vi "VirtualPowerPlantWithModelBasedFaultDetection(Giulio_v1).vi"() -> ()   [LabVIEW 2017]
uses:
  <vilib>/Platform/TimedLoop/XDataNode/timing_clust.ctl
  <vilib>/Platform/TimedLoop/XDataNode/nitl_modes.ctl
  <vilib>/Platform/TimedLoop/XDataNode/wakeup.ctl
  <vilib>/Utility/file.llb/Write Delimited Spreadsheet (string).vi
  <vilib>/Utility/file.llb/Write Delimited Spreadsheet (DBL).vi
  <vilib>/platform/TimedLoop/XDataNode/XDataNode.xnode
  <vilib>/express/express arith-compare/Formula/XNode/ExpressFormulaBlockNode.xnode
  <vilib>/Platform/TimedLoop/XDataNode/XDNodeRunTimeDep.lvlib
panel:
  out "Sensor 4":cluster{"placeholder1":dbl, dbl}(graph)
  out "Sensor 3":cluster{"placeholder1":dbl, dbl}(graph)
  out "Sensor 2":cluster{"placeholder1":dbl, dbl}(graph)
  out "Sensor 1":cluster{"placeholder1":dbl, dbl}(graph)
  in  "dTsamplethreshold":dbl=10.0
  in  "Tsamplethreshold":dbl=3.0
  in  "dTthreshold4":dbl=2.1702
  in  "dTthreshold3":dbl=2.8362
  in  "dTthreshold2":dbl=2.6736
  in  "dTthreshold1":dbl=2.361
  in  "Tthreshold4":dbl=0.4812
  in  "Tthreshold3":dbl
  in  "Tthreshold2":dbl=0.5934
  in  "Tthreshold1":dbl=0.588
  in  "Weight of measured values in filter":dbl=0.01
  in  "CTAH_control_on":dbl
  in  "CTAH_setpoint":dbl
  in  "CTAH_freq":dbl
  in  "P_in":dbl
  in  "T_wall placeholder":dbl
  in  "mdot":dbl
  out "Warnings":string
  in  "stop":bool
  in  "Measured Values":dbl
  out "Cold Leg Temp":dbl
  out "Primary HX Outlet Temp":dbl
  out "Hot Leg Temp":dbl
  out "color3":u32(colorbox)
  out "Heater Outlet Temp":dbl caption="C"
  out "color4":u32(colorbox)
  out "color2":u32(colorbox)
  in  "Upper Operating Pressure":dbl=6154480.5
  in  "Pump Efficiency":dbl=0.95
  in  "Turbine Efficiency":dbl=0.95
  in  "Pinch Point Temp Difference":dbl=15.0
  in  "Lower Operating Pressure":dbl=7093.0
  in  "Mass Flowrate":dbl=418.0
  in  "Pressure Drop in HX 2nd pass":dbl
  in  "Pressure Drop in HX 1st pass":dbl
  in  "LPT Work Output":dbl=137940000.0
  in  "HPT Work Output":dbl=1000000.0
  in  "LPT Efficiency":dbl=0.8
  in  "HPT Efficiency":dbl=0.8
  in  "Compressor Efficiency":dbl=0.7
  in  "LPT Expansion Ratio":dbl=5.13
  in  "Incoming Air Pressure":dbl=101325.0
  in  "HPT Expansion Ratio":dbl=3.77
  in  "Incoming Air Temp":dbl=298.0
  in  "Compression Ratio":dbl=19.6
  out "h_1":dbl
  out "R_T_1":dbl
  out "R_P_1":dbl
  out "h_6":dbl
  out "R_T_6":dbl
  out "R_P_6":dbl
  out "h_5":dbl
  out "R_T_5":dbl
  out "R_P_5":dbl
  out "h_4":dbl
  out "R_T_4":dbl
  out "R_P_4":dbl
  out "T_6":dbl
  out "P_6":dbl
  out "T_5":dbl
  out "P_5":dbl
  out "T_4":dbl
  out "P_4":dbl
  out "T_3":dbl
  out "P_3":dbl
  out "T_2":dbl
  out "P_2":dbl
  out "T_1":dbl
  out "P_1":dbl
  out "color1":u32(colorbox)
  # "Reactor Loop"
  # "Brayton Cycle"
  # "Rankine Cycle"
  # "ST"
  # "Compressor"
  # "HPT"
  # "LPT"
  # "Reactor"
  # "HRSG"
  # "Primary Heat\nExchanger"
  # "Condenser"
  # "Pump"
  # "Pump"
  # "Developer's Tools"
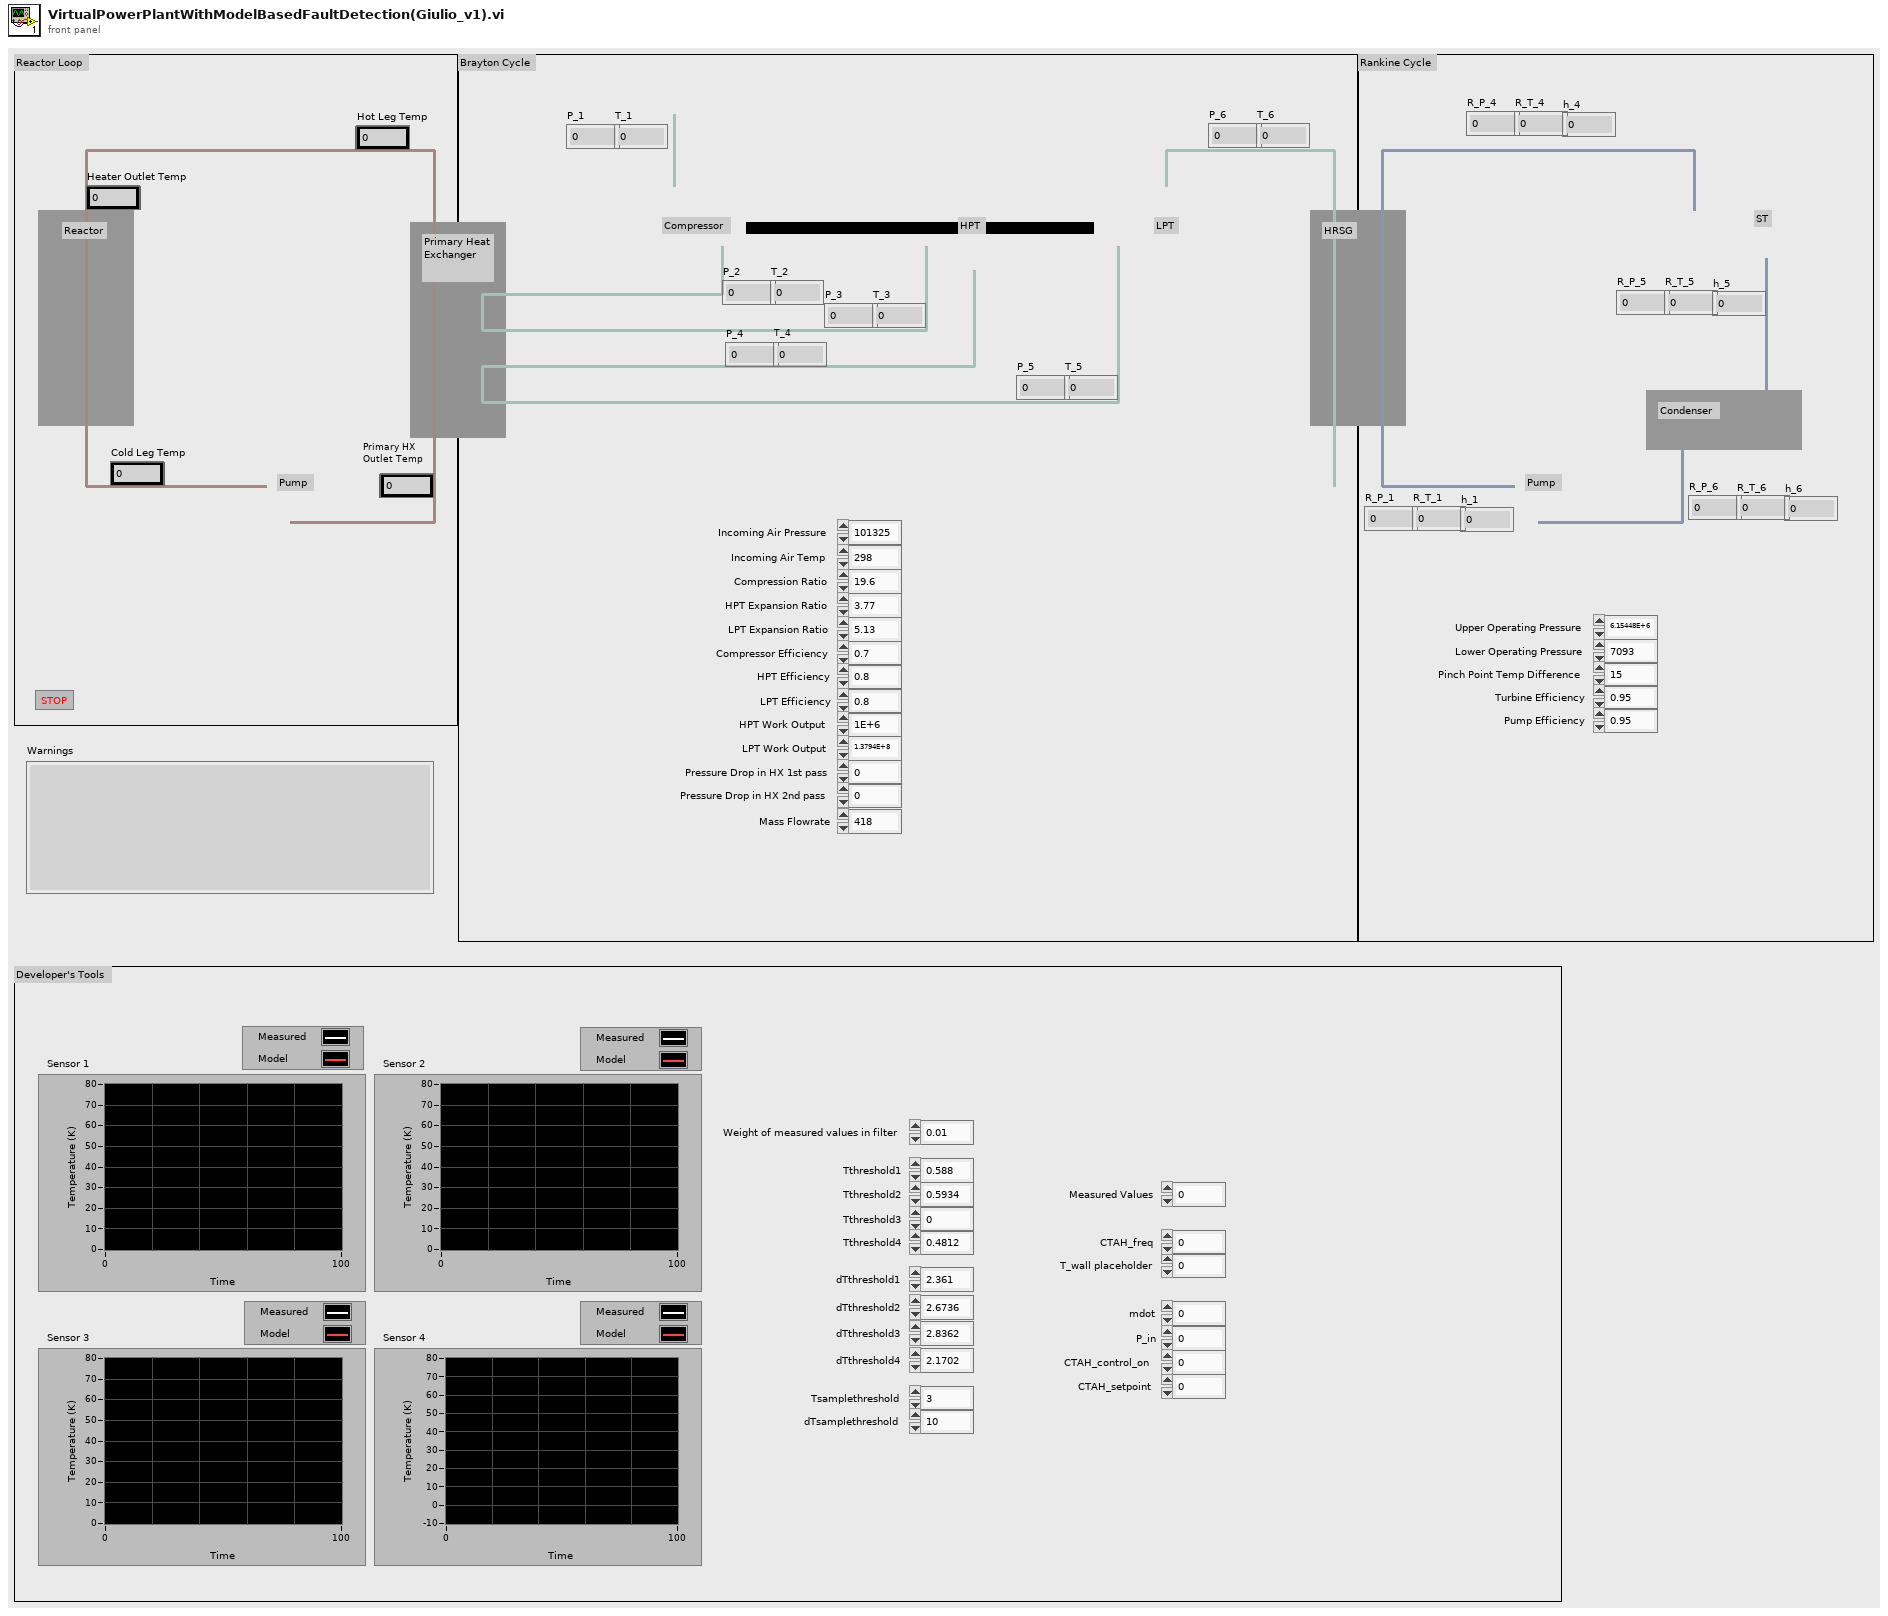
[diagram p1: front panel]
types:
  T1 = typedef "XDNodeRunTimeDep.lvlib/timing_clust.ctl" = cluster{"Expected End [f-1]":u64, "Actual End [f-1]":u64, "Finished Late? [f-1]":bool, "Expected End [i-1]":u64, "Actual End [i-1]":u64, "Finished Late? [i-1]":bool, "Expected Start [i]":u64, "Actual Start [i]":u64, "Expected Start [f]":u64, "Actual Start [f]":u64, "Source Name":string, "Structure Name":string, "Period":i64, "Deadline":i64, "Offset":i64, "Start":i64, "Priority":i32, "Timeout":i32, "Mode":T2, "Wakeup Reason":T3, "Error":errorcluster, "Source Type":string, "Secondary Source Type":string, "Global End Time":u64, "Global Start Time":u64, "Frame Duration":u64, "Iteration Duration":u64, "Assigned CPU":i32, "I/O Scan Engine Mode":u32}
  T2 = typedef "XDNodeRunTimeDep.lvlib/nitl_modes.ctl" = enum32{"No Change", "Process missed periods, maintain original phase", "Discard missed periods, maintain original phase", "Process missed periods, ignore original phase", "Discard missed periods, ignore original phase"}
  T3 = typedef "XDNodeRunTimeDep.lvlib/wakeup.ctl" = enum32{"Normal", "Aborted", "Asynchronous wakeup", "Timing source error", "Timed loop error", "Timeout"}
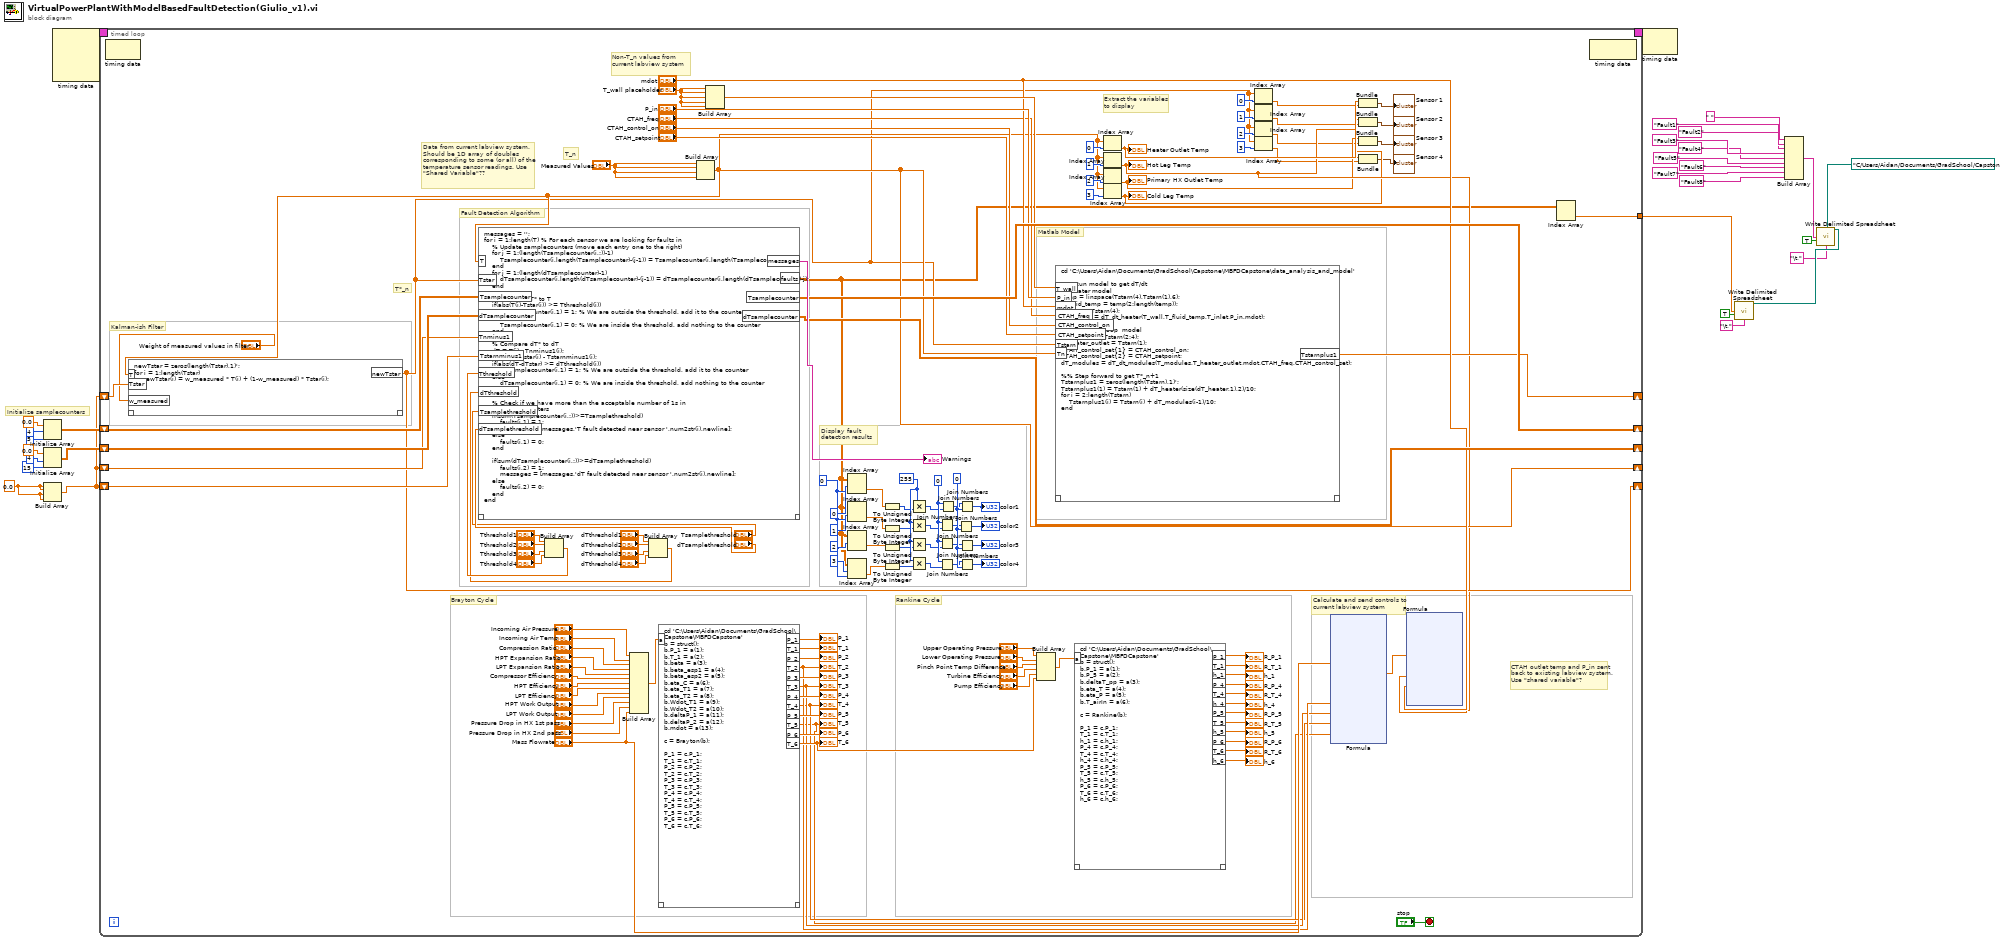
[diagram p0: block diagram]
diagram:
  w19 = 0.0
  # "Initialize samplecounters"
  n1 = Initialize Array(0.0, 4, 5) -> (w25:dbl[][])
  n2 = Initialize Array(0.0, 4, 15) -> (w24:dbl[][])
  n3 = Build Array(w19, w19, w19, w19) -> (w18:dbl[])
  n4 = node-c288() -> (w29:T1)  [unwired: 4 in]
  n5 = timed-loop {
    shift-right: [w93] -> _
    shift-left: w18 -> [w92]
    shift-right: [w105] -> _
    shift-left: w25 -> [w103]
    shift-right: [w104] -> _
    shift-left: w24 -> [w102]
    shift-right: [w91] -> _
    shift-left: w18 -> [w101]
    shift-right: [w44] -> _
    shift-left: w18 -> [w100]
    timing: w29 -> [_]
    timing-out: [_] -> w28
    tunnel: [w30] -> w17
    stop <- "stop" stop-if-true
    w61 = u8 255
    w62 = u8 0
    w63 = u8 0
    w68 = 0
    # "Kalman-ish Filter"
    # "Non-T_n values from current labview system"
    # "Extract the variables to display"
    # "T_n"
    # "Data from current labview system. Should be 1D array of doubles corresponding to some (or all) of the temperature sensor readings. Use \"Shared Variable\"??"
    # "CTAH outlet temp and P_in sent back to existing labview system. Use \"shared variable\"?"
    # "Calculate and send controls to current labview system"
    # "Display fault detection results"
    # "Fault Detection Algorithm"
    # "T*_n"
    # "Matlab Model"
    # "Rankine Cycle"
    # "Brayton Cycle"
    n6 = node-c288() -> ()  [unwired: 1 in, 1 out]
    n7 = Build Array("Tthreshold1", "Tthreshold2", "Tthreshold3", "Tthreshold4") -> (w85:dbl[])
    n8 = Build Array("Incoming Air Pressure", "Incoming Air Temp", "Compression Ratio", "HPT Expansion Ratio", "LPT Expansion Ratio", "Compressor Efficiency", "HPT Efficiency", "LPT Efficiency", "HPT Work Output", "LPT Work Output", "Pressure Drop in HX 1st pass", "Pressure Drop in HX 2nd pass", "Mass Flowrate") -> (w145:dbl[])
    n9 = Build Array("dTthreshold1", "dTthreshold2", "dTthreshold3", "dTthreshold4") -> (w80:dbl[])
    n10 = script code="cd 'C:\\Users\\Aidan\\Documents\\GradSchool\\Capstone\\MBFDCapstone'\nb = struct();\nb.P_1 = a(1);\nb.T_1 = a(2);\nb.beta = a(3);\nb.beta_esp1 = a(4);\nb.beta_esp2 = a(5);\nb.eta_C = a(6);\nb.eta_T1 = a(7);\nb.eta_T2 = a(8);\nb.Wdot_T1 = a(9);\nb.Wdot_T2 = a(10);\nb.deltaP_1 = a(11);\nb.deltaP_2 = a(12);\nb.mdot = a(13);\n\nc = Brayton(b);\n\nP_1 = c.P_1;\nT_1 = c.T_1;\nP_2 = c.P_2;\nT_2 = c.T_2;\nP_3 = c.P_3;\nT_3 = c.T_3;\nP_4 = c.P_4;\nT_4 = c.T_4;\nP_5 = c.P_5;\nT_5 = c.T_5;\nP_6 = c.P_6;\nT_6 = c.T_6;"("a"=w145) -> ("P_1"=→"P_1":dbl, "T_1"=→"T_1":dbl, "P_2"=→"P_2":dbl, "T_2"=w110:dbl, "P_3"=→"P_3":dbl, "T_3"=w109:dbl, "P_4"=→"P_4":dbl, "T_4"=w108:dbl, "P_5"=→"P_5":dbl, "T_5"=w107:dbl, "P_6"=→"P_6":dbl, "T_6"=w131:dbl)  [unwired: 1 in, 1 out]
    "T_2" <- w110
    "T_3" <- w109
    "T_4" <- w108
    "T_5" <- w107
    "T_6" <- w131
    n11 = Build Array("Measured Values", "Measured Values", "Measured Values", "Measured Values") -> (w91:dbl[])
    n12 = script code="newTstar = zeros(length(Tstar),1)';\nfor i = 1:length(Tstar)\n    newTstar(i) = w_measured * T(i) + (1-w_measured) * Tstar(i);\nend"("T"=w91, "Tstar"=w92, "w_measured"="Weight of measured values in filter") -> ("newTstar"=w44:dbl[])  [unwired: 1 in, 1 out]
    n13 = script code="messages = '';\nfor i = 1:length(T) % For each sensor we are looking for faults in\n    % Update samplecounters (move each entry one to the right)\n    for j = 1:(length(Tsamplecounter(i,:))-1)\n        Tsamplecounter(i,length(Tsamplecounter)-(j-1)) = Tsamplecounter(i,length(Tsamplecounter)-j);\n    end\n    for j = 1:(length(dTsamplecounter)-1)\n        dTsamplecounter(i,length(dTsamplecounter)-(j-1)) = dTsamplecounter(i,length(dTsamplecounter)-j);\n    end\n\n    % Compare T* to T\n    if(abs(T(i)-Tstar(i)) >= Tthreshold(i))\n        Tsamplecounter(i,1) = 1; % We are outside the threshold, add it to the counter\n    else\n        Tsamplecounter(i,1) = 0; % We are inside the threshold, add nothing to the counter\n    end\n    \n    % Compare dT* to dT\n    dT = T(i) - Tnminus1(i);\n    dTstar = Tstar(i) - Tstarnminus1(i);\n    if(abs(dT-dTstar) >= dTthreshold(i))\n        dTsamplecounter(i,1) = 1; % We are outside the threshold, add it to the counter\n    else\n        dTsamplecounter(i,1) = 0; % We are inside the threshold, add nothing to the counter\n    end\n    \n    % Check if we have more than the acceptable number of 1s in\n    % samplecounters\n    if(sum(Tsamplecounter(i,:))>=Tsamplethreshold)\n        faults(i,1) = 1;\n        messages = [messages,'T fault detected near sensor ',num2str(i),newline];\n    else\n        faults(i,1) = 0;\n    end\n       \n    if(sum(dTsamplecounter(i,:))>=dTsamplethreshold)\n        faults(i,2) = 1;\n        messages = [messages,'dT fault detected near sensor ',num2str(i),newline];\n    else\n        faults(i,2) = 0;\n    end\nend"("T"=w91, "Tstar"=w44, "Tsamplecounter"=w103, "dTsamplecounter"=w102, "Tnminus1"=w101, "Tstarnminus1"=w100, "Tthreshold"=w85, "dTthreshold"=w80, "Tsamplethreshold"="Tsamplethreshold", "dTsamplethreshold"="dTsamplethreshold") -> ("faults"=w31:dbl[][], "messages"=→"Warnings":string, "Tsamplecounter"=w105:dbl[][], "dTsamplecounter"=w104:dbl[][])  [unwired: 1 in, 1 out]
    n14 = Build Array("T_wall placeholder", "T_wall placeholder", "T_wall placeholder", "T_wall placeholder", "T_wall placeholder") -> (w99:dbl[])
    n15 = Index Array(array=w31, index (row)=0, index (col)=w68) -> (element=w64:dbl)
    n16 = Index Array(array=w31, index (row)=1, index (col)=w68) -> (element=w65:dbl)
    n17 = Index Array(array=w31, index (row)=2, index (col)=w68) -> (element=w66:dbl)
    n18 = Index Array(array=w31, index (row)=3, index (col)=w68) -> (element=w67:dbl)
    n19 = To Unsigned Byte Integer(number=w64) -> (unsigned 8bit integer=w60:u8)
    n20 = To Unsigned Byte Integer(number=w65) -> (unsigned 8bit integer=w58:u8)
    n21 = To Unsigned Byte Integer(number=w66) -> (unsigned 8bit integer=w56:u8)
    n22 = To Unsigned Byte Integer(number=w67) -> (unsigned 8bit integer=w54:u8)
    n23 = Multiply(x=w61, y=w60) -> (x*y=w59:u8)
    n24 = Multiply(x=w61, y=w58) -> (x*y=w57:u8)
    n25 = Multiply(x=w61, y=w56) -> (x*y=w55:u8)
    n26 = Multiply(x=w61, y=w54) -> (x*y=w53:u8)
    n27 = Join Numbers(hi=w62, lo=w57) -> ((hi.lo)=w50:u16)
    n28 = Join Numbers(hi=w62, lo=w55) -> ((hi.lo)=w51:u16)
    n29 = Join Numbers(hi=w62, lo=w53) -> ((hi.lo)=w52:u16)
    n30 = Join Numbers(hi=w62, lo=w59) -> ((hi.lo)=w49:u16)
    n31 = Join Numbers(hi=w50, lo=w63) -> ((hi.lo)=→"color2":u32)
    n32 = Join Numbers(hi=w49, lo=w63) -> ((hi.lo)=→"color1":u32)
    n33 = Join Numbers(hi=w51, lo=w63) -> ((hi.lo)=→"color3":u32)
    n34 = Join Numbers(hi=w52, lo=w63) -> ((hi.lo)=→"color4":u32)
    n35 = Build Array("Upper Operating Pressure", "Lower Operating Pressure", "Pinch Point Temp Difference", "Turbine Efficiency", "Pump Efficiency", w131) -> (w132:dbl[])
    n36 = script code="cd 'C:\\Users\\Aidan\\Documents\\GradSchool\\Capstone\\MBFDCapstone\\data_analysis_and_model'\n\n%% Run model to get dT/dt\n% Heater model\ntemp = linspace(Tstarn(4),Tstarn(1),6);\nT_fluid_temp = temp(2:length(temp));\nT_inlet = Tstarn(4);\ndT_heater = dT_dt_heater(T_wall,T_fluid_temp,T_inlet,P_in,mdot);\n\n% Rest of the loop  model\nT_modules = Tstarn(2:4);\nT_heater_outlet = Tstarn(1);\nCTAH_control_set{1} = CTAH_control_on;\nCTAH_control_set{2} = CTAH_setpoint;\ndT_modules = dT_dt_modules(T_modules,T_heater_outlet,mdot,CTAH_freq,CTAH_control_set);\n\n%% Step forward to get T*_n+1\nTstarnplus1 = zeros(length(Tstarn),1)';\nTstarnplus1(1) = Tstarn(1) + dT_heater(size(dT_heater,1),2)/10;\nfor i = 2:length(Tstarn)\n    Tstarnplus1(i) = Tstarn(i) + dT_modules(i-1)/10;\nend"("Tstarn"=w44, "T_wall"=w99, "P_in"="P_in", "mdot"="mdot", "Tn"=w91, "CTAH_freq"="CTAH_freq", "CTAH_control_on"="CTAH_control_on", "CTAH_setpoint"="CTAH_setpoint") -> ("Tstarnplus1"=w93:dbl[])  [unwired: 1 in, 1 out]
    n37 = script code="cd 'C:\\Users\\Aidan\\Documents\\GradSchool\\Capstone\\MBFDCapstone'\nb = struct();\nb.P_1 = a(1);\nb.P_5 = a(2);\nb.deltaT_pp = a(3);\nb.eta_T = a(4);\nb.eta_P = a(5);\nb.T_airIn = a(6);\n\nc = Rankine(b);\n\nP_1 = c.P_1;\nT_1 = c.T_1;\nh_1 = c.h_1;\nP_4 = c.P_4;\nT_4 = c.T_4;\nh_4 = c.h_4;\nP_5 = c.P_5;\nT_5 = c.T_5;\nh_5 = c.h_5;\nP_6 = c.P_6;\nT_6 = c.T_6;\nh_6 = c.h_6;"("a"=w132) -> ("P_1"=→"R_P_1":dbl, "T_1"=→"R_T_1":dbl, "h_1"=→"h_1":dbl, "P_4"=→"R_P_4":dbl, "T_4"=→"R_T_4":dbl, "h_4"=→"h_4":dbl, "P_5"=→"R_P_5":dbl, "T_5"=→"R_T_5":dbl, "h_5"=→"h_5":dbl, "P_6"=→"R_P_6":dbl, "T_6"=→"R_T_6":dbl, "h_6"=→"h_6":dbl)  [unwired: 1 in, 1 out]
    n38 = Index Array(array=w91, index=0) -> (element=w43:dbl)
    "Heater Outlet Temp" <- w43
    n39 = Index Array(array=w91, index=1) -> (element=w42:dbl)
    "Hot Leg Temp" <- w42
    n40 = Index Array(array=w91, index=2) -> (element=w41:dbl)
    "Primary HX Outlet Temp" <- w41
    n41 = Index Array(array=w91, index=3) -> (element=w40:dbl)
    "Cold Leg Temp" <- w40
    n42 = Index Array(array=w44, index=0) -> (element=w39:dbl)
    n43 = Index Array(array=w44, index=1) -> (element=w38:dbl)
    n44 = Index Array(array=w44, index=2) -> (element=w37:dbl)
    n45 = Index Array(array=w44, index=3) -> (element=w36:dbl)
    n46 = xnode "Formula"("mdot"="Mass Flowrate", "T2"=w110, "T3"=w109, "T4"=w108, "T5"=w107) -> ("Result"=w106:dbl)  [unwired: 1 in, 1 out]
    n47 = Bundle("Measured Values"=w43, w39) -> (→"Sensor 1":cluster{"Measured Values":dbl, dbl})  [unwired: 1 in]
    n48 = Bundle("Measured Values"=w42, w38) -> (→"Sensor 2":cluster{"Measured Values":dbl, dbl})  [unwired: 1 in]
    n49 = Bundle("Measured Values"=w41, w37) -> (→"Sensor 3":cluster{"Measured Values":dbl, dbl})  [unwired: 1 in]
    n50 = Bundle("Measured Values"=w40, w36) -> (→"Sensor 4":cluster{"Measured Values":dbl, dbl})  [unwired: 1 in]
    n51 = xnode "Formula"("Pout"=w106, "Tin"=w42, "mdot"="mdot") -> ()  [unwired: 2 in, 2 out]
    n52 = Index Array(array=w31) -> (element=w30:dbl[])  [unwired: 2 in]
    n53 = node-c288() -> ()  [unwired: 1 in, 1 out]
  }
  n54 = node-c288(w28) -> ()  [unwired: 1 out]
  n55 = Build Array(" ", "Fault1", "Fault2", "Fault3" ("element"), "Fault4" ("element"), "Fault5" ("element"), "Fault6" ("element"), "Fault7" ("element"), "Fault8" ("element")) -> (w1:string[])
  n56 = call-poly <vilib>:"Write Delimited Spreadsheet.vi"("file path (dialog if empty)"=path "C:/Users/Aidan/Documents/GradSchool/Capstone/MBFDCapstone/data_analysis_and_model", "1D data"=w1, "append to file? (new file:F)"=TRUE, "delimiter (\\t)"="\t," ("delimiter (\\t)")) -> ("new file path (Not A Path if cancelled)"=w13:path)  [unwired: 10 in, 1 out]
  n57 = call-poly <vilib>:"Write Delimited Spreadsheet.vi"("file path (dialog if empty)"=w13, "1D data"=w17, "append to file? (new file:F)"=TRUE, "delimiter (\\t)"="\t," ("delimiter (\\t)")) -> ()  [unwired: 10 in, 2 out]
